vi "Agilent U2722 - Current output.vi"() -> ()   [LabVIEW 2010]
doc: "This example shows how to configure the instrument's output voltage level, over current protection, and over voltage protection. The actual voltage level and actual current level are returned as well as whether over voltage protection (OVP) or over current protection (OCP) has been tripped."
uses:
  Agilent U2722.lvlib
panel:
  in  "Output Level (mA)":dbl=1.0
  in  "Channel (1: Channel 1)":u16(ring)=1 items=["Channel 1"=1, "Channel 2"=2, "Channel 3"=3]
  in  "Stop Output":bool
  out "Actual Current Limit (A)":dbl format="%.2f"
  out "Actual Voltage Level (V)":dbl format="%.2f"
  in  "VISA resource name":refnum<visa-resource-name>
  # "(c) 2009 National Instruments.  ALL RIGHTS RESERVED."
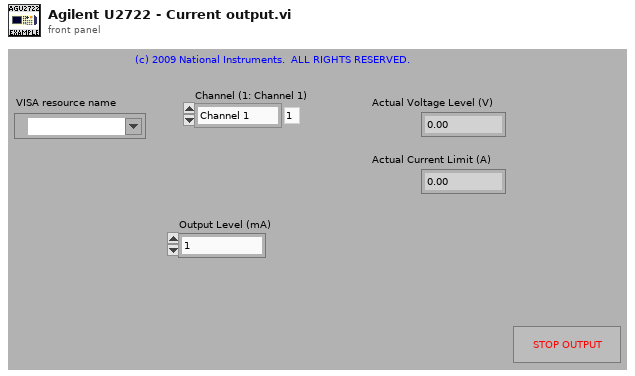
[diagram p1: front panel]
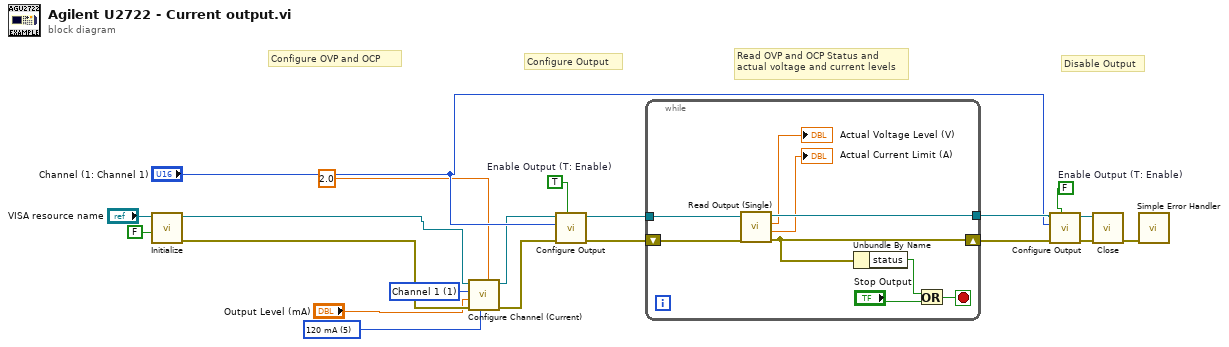
[diagram p0: block diagram]
diagram:
  w2 = u16 5 items=["1 uA", "10 uA", "100 uA", "1 mA", "10 mA", "120 mA"] ("Current Range (0: 1 uA)")
  w4 = u16 1 items=["Channel 1"=1, "Channel 2"=2, "Channel 3"=3] ("Channel (1: Channel 1)")
  w18 = TRUE  # Enable Output (T: Enable)
  w11 = FALSE  # Enable Output (T: Enable)
  # "Disable Output"
  # "Read OVP and OCP Status and\nactual voltage and current levels"
  # "Configure Output"
  # "Configure OVP and OCP"
  n1 = call "Initialize.vi"("ID Query (True)"=FALSE, "VISA resource name"="VISA resource name") -> ("error out"=w7:errorcluster, "VISA resource name out"=w8:refnum<visa-resource-name>)  [unwired: 8 in]
  n2 = call "Configure Channel (Current).vi"("Voltage Limit (2.0 V)"=2.0 ("Voltage Limit"), "Current Range (0: 1 uA)"=w2, "error in (no error)"=w7, "Output Level (1.0 mA)"="Output Level (mA)", "Channel (1: Channel 1)"=w4, "VISA resource name"=w8) -> ("error out"=w5:errorcluster, "VISA resource name out"=w6:refnum<visa-resource-name>)  [unwired: 4 in]
  n3 = call "Configure Output.vi"("Enable Output (T: Enable)"=w18, "error in (no error)"=w5, "Channel (1: Channel 1)"="Channel (1: Channel 1)", "VISA resource name"=w6) -> ("error out"=w16:errorcluster, "VISA resource name out"=w17:refnum<visa-resource-name>)  [unwired: 6 in]
  n4 = while {
    tunnel: w17 -> [w27]
    shift-right: [w22] -> w14
    shift-left: w16 -> [w26]
    tunnel: [w25] -> w15
    stop <- w29 stop-if-true
    n5 = call "Read Output (Single).vi"("error in (no error)"=w26, "VISA resource name"=w27) -> ("error out"=w22:errorcluster, "Actual Current Level (A)"=→"Actual Current Limit (A)":dbl, "Actual Voltage Level (V)"=→"Actual Voltage Level (V)":dbl, "VISA resource name out"=w25:refnum<visa-resource-name>)  [unwired: 6 in]
    n6 = Unbundle By Name(w22) -> ("status"=w21:bool)
    n7 = Or(x=w21, y="Stop Output") -> (x .or. y?=w29:bool)
  }
  n8 = call "Configure Output.vi"("Enable Output (T: Enable)"=w11, "error in (no error)"=w14, "Channel (1: Channel 1)"="Channel (1: Channel 1)", "VISA resource name"=w15) -> ("error out"=w12:errorcluster, "VISA resource name out"=w13:refnum<visa-resource-name>)  [unwired: 6 in]
  n9 = call "Close.vi"("error in (no error)"=w12, "VISA resource name"=w13) -> ("error out"=w20:errorcluster)  [unwired: 9 in]
  n10 = call <vilib>:"Simple Error Handler.vi"("error in (no error)"=w20) -> ()  [unwired: 4 in, 5 out]
